vi "getFingerprint.vi"(0 "HGF_GPG in":refnum<class "HGF_GPG.lvclass">, 1 "options file":path, 2 "keyringfile":path, 3 "Sec keyringfile":path, 5 "error in (no error)":errorcluster, 6 "key-id":string, 8 "Trust DB":path) -> (10 "dup Trust DB":path, 12 "fingerprint":string, 14 "dup HGF_GPG":refnum<class "HGF_GPG.lvclass">, 15 "dup options file":path, 16 "dup keyringfile":path, 17 "dup Sec keyringfile":path, 19 "error out":errorcluster)   [LabVIEW 2012, in "HGF_GPG.lvlib" / "HGF_GPG.lvclass"]
doc: "Get fingerprint of Key-ID. If no Key-ID is set, the Objects Fingerprint will be returned."
uses:
  HGF_GPG.lvclass
  HGF_GPG.lvclass/HGF_GPG.ctl
  <vilib>/regexp/Match Regular Expression.xnode
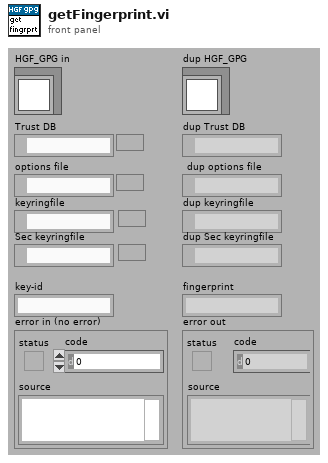
[diagram p1: front panel]
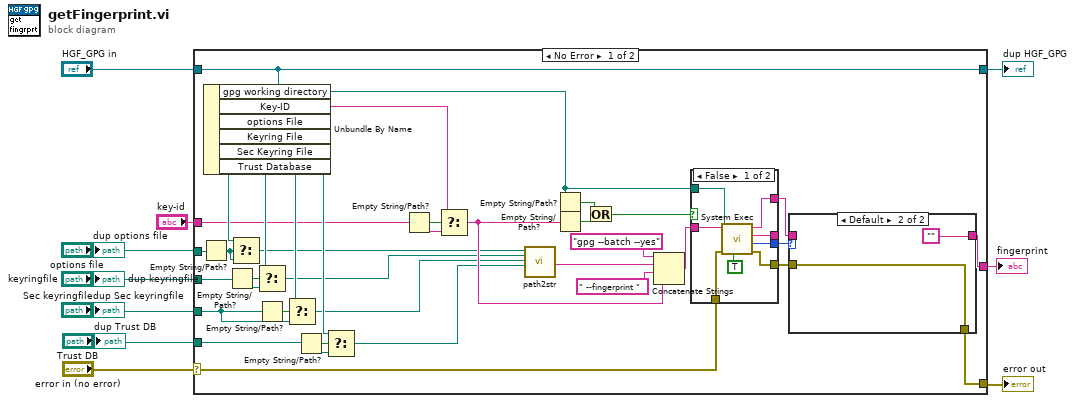
[diagram p0: block diagram]
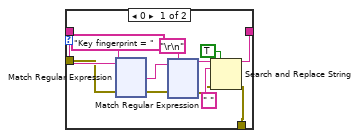
[diagram p2: hidden frame]
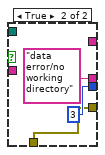
[diagram p3: hidden frame]
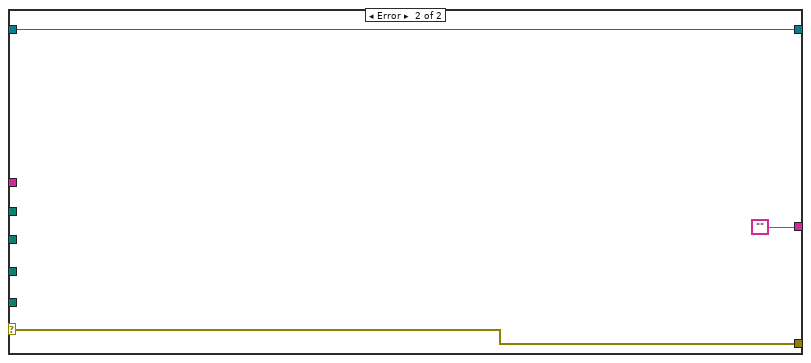
[diagram p4: hidden frame]
diagram:
  n1 = case shown="No Error" "error in (no error)" {
    selector: "error in (no error)" -> [w31 w295]
    tunnel: [w27 w295] -> w10
    tunnel: [w41 w294] -> w8
    tunnel: "HGF_GPG in" -> [w41 w294]
    tunnel: "key-id" -> [w38 _]
    tunnel: [w29 ""] -> w6
    tunnel: "options file" -> [w21 _]
    tunnel: "keyringfile" -> [w18 _]
    tunnel: "Sec keyringfile" -> [w15 _]
    tunnel: "Trust DB" -> [w12 _]
    frame No Error {
      n2 = Empty String/Path?(string/path=w21) -> (empty?=w22:bool)
      n3 = Unbundle By Name(w41) -> ("gpg working directory"=w34:path, "Key-ID"=w39:string, "options File"=w42:path, "Keyring File"=w43:path, "Sec Keyring File"=w45:path, "Trust Database"=w44:path)
      n4 = Empty String/Path?(string/path=w18) -> (empty?=w19:bool)
      n5 = Select(t=w42, s=w22, f=w21) -> (s? t:f=w20:path)
      n6 = Select(t=w43, s=w19, f=w18) -> (s? t:f=w16:path)
      n7 = Empty String/Path?(string/path=w15) -> (empty?=w17:bool)
      n8 = Select(t=w45, s=w17, f=w15) -> (s? t:f=w13:path)
      n9 = Empty String/Path?(string/path=w12) -> (empty?=w14:bool)
      n10 = Select(t=w44, s=w14, f=w12) -> (s? t:f=w11:path)
      n11 = Empty String/Path?(string/path=w38) -> (empty?=w40:bool)
      n12 = Select(t=w39, s=w40, f=w38) -> (s? t:f=w24:string)
      n13 = call "path2str.vi"("options file"=w20, "keyringfile"=w16, "Sec keyringfile"=w13, "Trust DB"=w11) -> ("opt/keyr/seckeyr/trusdb"=w23:string)  [unwired: 2 in, 13 out]
      n14 = Empty String/Path?(string/path=w34) -> (empty?=w37:bool)
      n15 = Empty String/Path?(string/path=w24) -> (empty?=w36:bool)
      n16 = Or(x=w37, y=w36) -> (x .or. y?=w35:bool)
      n17 = Concatenate Strings("gpg --batch --yes", w23, " --fingerprint " ("string"), w24) -> (w32:string)
      n18 = case shown="False" w35 {
        tunnel: w31 -> [w288 w290]
        tunnel: w34 -> [w287 _]
        tunnel: w32 -> [w286 _]
        tunnel: [w285 _] -> w26
        tunnel: [w284 "data error/no working directory" ("standard error")] -> _
        tunnel: [w283 3 ("return code")] -> w30
        tunnel: [w282 w290] -> w28
        frame False {
          n19 = call <vilib>:"System Exec.vi"("run minimized? (F)"=TRUE, "error in (no error)"=w288, "working directory"=w287, "command line"=w286) -> ("error out"=w282:errorcluster, "return code"=w283:i32, "standard error"=w284:string, "standard output"=w285:string)  [unwired: 2 in, 2 out]
        }
        frame True {
        }
      }
      n20 = case shown="Default" w30 {
        tunnel: w26 -> [w52 _]
        tunnel: [w51 ""] -> w29
        tunnel: w28 -> [w50 w280]
        tunnel: [w47 w280] -> w27
        frame 0 {
          n21 = xnode "Match Regular Expression"("input string"=w52, "regular expression"="Key fingerprint = ", "error in"=w50) -> ("after match"=w54:string, "error out"=w49:errorcluster)  [unwired: 1 in, 5 out]
          n22 = xnode "Match Regular Expression"("input string"=w54, "regular expression"="\r\n", "error in"=w49) -> ("before match"=w55:string, "error out"=w48:errorcluster)  [unwired: 1 in, 5 out]
          n23 = Search and Replace String(replace all?=TRUE ("replace all? (F)"), input string=w55, search string=" ", error in=w48) -> (result string=w51:string, error out=w47:errorcluster)  [unwired: 6 out]
        }
        frame Default {
        }
      }
    }
    frame Error {
    }
  }
  "error out" <- w10
  "dup HGF_GPG" <- w8
  "fingerprint" <- w6
  "dup keyringfile" <- "keyringfile"
  "dup options file" <- "options file"
  "dup Sec keyringfile" <- "Sec keyringfile"
  "dup Trust DB" <- "Trust DB"
